vi "Pre Launch Init.vi"(11 "Command Processor Actor in":refnum<class "Command Processor Actor.lvclass">) -> (0 "error out":errorcluster, 3 "Command Processor Actor out":refnum<class "Command Processor Actor.lvclass">)   [LabVIEW 2014, in "Robot Actor Framework.lvlib" / "Command Processor Actor.lvlib" / "Command Processor Actor.lvclass"]
doc: "(<B>Filename</B>: Actor Framework.lvlib:Actor.lvclass:Pre Launch Init.vi)\n\nDefines behavior that occurs after the Launch Nested Actor method is invoked but before the actor's Actor Core method begins running.\n\nBy default, this method does nothing. A descendant class may override it to define behavior."
uses:
  Command Processor Actor.lvclass
  Command Actor/Command Actor Class/Command Actor.lvclass
  Command Processor Actor.lvclass/Command Processor Actor.ctl
  <vilib>/ni/Actors/State Actor/State Actor/State Actor.lvclass
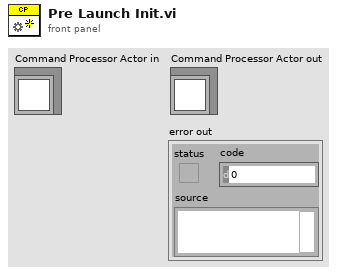
[diagram p1: front panel]
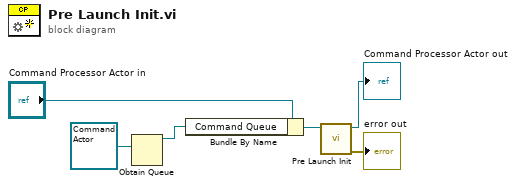
[diagram p0: block diagram]
diagram:
  n1 = Obtain Queue(element data type=refnum<class "Command Actor.lvclass"> refnum ("Robot Actor Framework.lvlib:Command Actor.lvlib:Command Actor.lvclass")) -> (queue out=w1:refnum<queue>)  [unwired: 4 in, 2 out]
  n2 = Bundle By Name(cluster="Command Processor Actor in", "Command Queue"=w1) -> (w2:refnum<class "Command Processor Actor.lvclass">)
  n3 = call-parent "Pre Launch Init.vi"("Actor in"=w2) -> ("error out"=→"error out":errorcluster, "Actor out"=→"Command Processor Actor out":refnum<class "Command Processor Actor.lvclass">)  [unwired: 9 in]
